vi "VSI Flash Write Bytes.vi"(6 "WriteLen":u16, 7 "pWriteData":u8[](array[numeric])=array[10240 elements], 9 "PageAddr":i32, 10 "DevIndex":i32, 11 "DevType":i32) -> (3 "function return":i32)   [LabVIEW 2010, in "ControlSPI.lvlib"]
doc: "int WINAPI VSI_FlashWriteBytes(int DevType,int DevIndex,int PageAddr,unsigned char *pWriteData,unsigned short WriteLen);"
uses:
  ControlSPI.lvlib
  ControlSPI/Ginkgo_Driver.dll
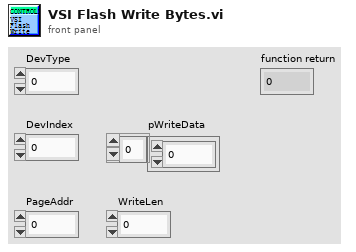
[diagram p1: front panel]
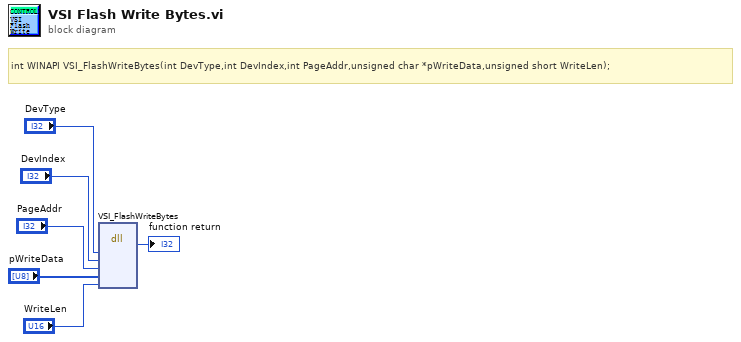
[diagram p0: block diagram]
diagram:
  # "int WINAPI VSI_FlashWriteBytes(int DevType,int DevIndex,int PageAddr,unsigned char *pWriteData,unsigned short WriteLen);"
  n1 = dll-call lib="E:/Project/vt_ginkgo/truck/Ginkgo Driver/vs2010/Ginkgo_USB-I2C&SPI&CAN_API_v2.0.3.3/lib/labview_32bit/ControlSPI/Ginkgo_Driver.*" fn="VSI_FlashWriteBytes"("DevType"="DevType", "DevIndex"="DevIndex", "PageAddr"="PageAddr", "pWriteData"="pWriteData", "WriteLen"="WriteLen") -> (→"function return":i32)  [unwired: 8 in, 2 out]
